vi "Array Average.vi"(1 "Array to Average":dbl[](array[numeric])) -> (0 "Average":dbl)   [LabVIEW 2014, in "Linear Regression.lvlib"]
uses:
  Labview Reliability Implementation/Linear Regression/Linear Regression.lvlib
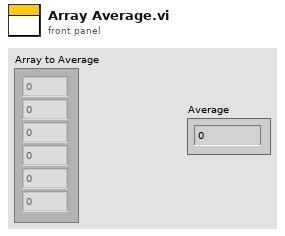
[diagram p1: front panel]
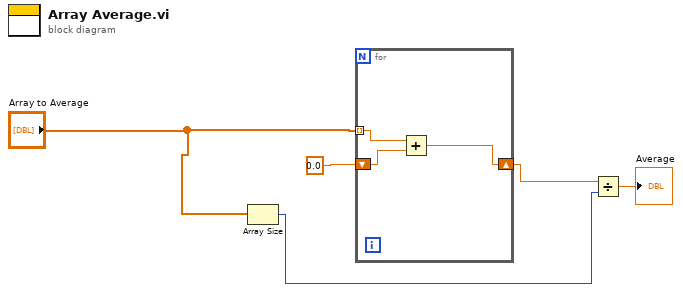
[diagram p0: block diagram]
diagram:
  n1 = Array Size(array="Array to Average") -> (size(s)=w3:i32)
  n2 = for {
    tunnel: "Array to Average" -> [w8] mode=indexing
    shift-right: [w6] -> w4
    shift-left: 0.0 -> [w7]
    n3 = Add(x=w8, y=w7) -> (x+y=w6:dbl)
  }
  n4 = Divide(x=w4, y=w3) -> (x/y=→"Average":dbl)
